vi "Measurement Parser.vi"(8 "error in (no error)":errorcluster, 9 "Universal Power Meter.lvlib:Universal Card.lvclass":refnum<class "Universal Card.lvclass">, 10 "Data Array":dbl[](array[numeric]), 11 "Universal Power Meter in":refnum<class "Universal Power Meter.lvclass">) -> (0 "error out":errorcluster, 2 "Waveform Graph":dynamicdata(graph), 3 "Universal Power Meter out":refnum<class "Universal Power Meter.lvclass">)   [LabVIEW 2013, in "Universal Power Meter.lvlib" / "Universal Power Meter.lvclass"]
uses:
  Universal Power Meter.lvclass
  Universal Card Class/Universal Card.lvclass
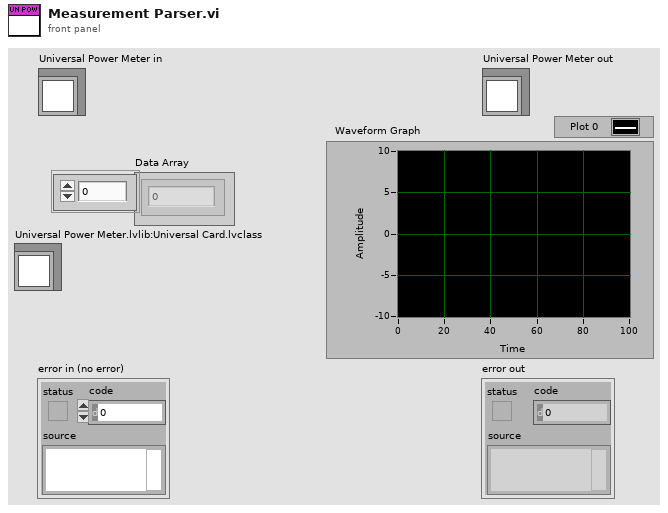
[diagram p1: front panel]
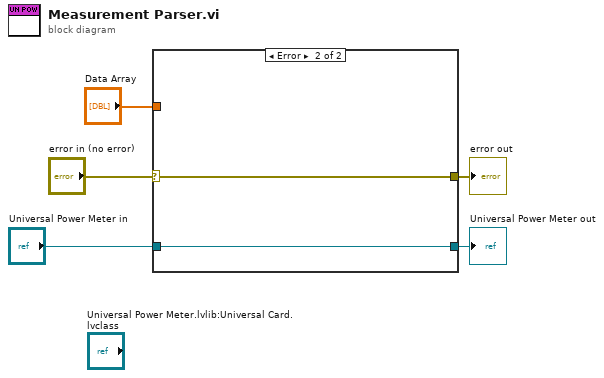
[diagram p0: block diagram]
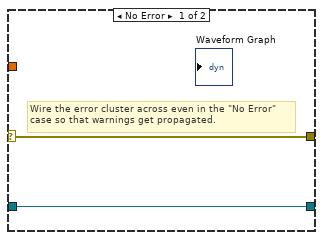
[diagram p2: hidden frame]
diagram:
  n1 = case shown="Error" "error in (no error)" {
    selector: "error in (no error)" -> [w6 w9]
    tunnel: [w6 w9] -> w4
    tunnel: [w7 w8] -> w2
    tunnel: "Universal Power Meter in" -> [w7 w8]
    tunnel: "Data Array" -> [_ _]
    frame No Error {
      # "Wire the error cluster across even in the \"No Error\"\ncase so that warnings get propagated."
    }
    frame Error {
    }
  }
  "error out" <- w4
  "Universal Power Meter out" <- w2
